vi "Pulse Parameters.vi"(0 "T1 Pulse Sequence":T19={"Preliminary Settings"={"Nº of Scans (ns)"=3, "Pulse Frequency"=10000000.0, "Nº of Vd"=3}, "Pulse Settings"={"Duration Signal P2"=20.0, "Power Level P2"=1023, "Phase P2"=90, "P2 Unit"=0, "Duration Signal P1"=20.0, "Power Level P1"=1023, "Phase P1"=90, "P1 Unit"=0}, "Acquisition Settings"={"Number Samples"=2000, "Time Between Points"=0.0, "Unit"=0}, "Delay Settings"={"Delay d1"=10.0, "Delay d2"=0.0, "d1 Unit"=0, "d2 Unit"=0, "Delay d30"=0.0, "d30 Unit"=0, "Vd Unit"=0, "Vd Values"="0"}} {"Delay Settings"."Vd Unit" items=["us", "ms"]; "Delay Settings"."d30 Unit" items=["us", "ms"]; "Delay Settings"."Delay d30" min=0.0 step=1.0; "Delay Settings"."d2 Unit" items=["us", "ms"]; "Delay Settings"."d1 Unit" items=["us", "ms"]; "Delay Settings"."Delay d2" min=0.0 step=1.0 format="%#_4g"; "Delay Settings"."Delay d1" min=0.0 step=1.0 format="%#_4g"; "Acquisition Settings"."Unit" items=["us", "ms"]; "Acquisition Settings"."Time Between Points" min=0.0 step=1.0; "Acquisition Settings"."Number Samples" step=1; "Pulse Settings"."P1 Unit" items=["us", "ms"]; "Pulse Settings"."Phase P1" max=270 step=90; "Pulse Settings"."Power Level P1" max=1023 step=1; "Pulse Settings"."Duration Signal P1" min=0.0 step=1.0 format="%#_4g"; "Pulse Settings"."P2 Unit" items=["us", "ms"]; "Pulse Settings"."Phase P2" max=270 step=90; "Pulse Settings"."Power Level P2" max=1023 step=1; "Pulse Settings"."Duration Signal P2" min=0.0 step=1.0 format="%#_4g"; "Preliminary Settings"."Nº of Vd" step=1; "Preliminary Settings"."Pulse Frequency" min=1.0 max=200000000.0 step=1000000.0 format="%^#_6e"; "Preliminary Settings"."Nº of Scans (ns)" step=1}, 1 "action":T20, 5 "90 Degree Pulse Sequence":T18={"Delay Settings"={"Delay d1"=10.0, "Delay d2"=0.0, "d1 Unit"=0, "d2 Unit"=0}, "Preliminary Settings"={"Nº of Scans (ns)"=3, "Pulse Frequency"=10000000.0}, "Pulse Settings"={"Duration Signal P1"=20.0, "Power Level"=1023, "Phase"=90, "P1 Units"=0}, "Acquisition Settings"={"Number Samples"=2000, "Time Between Points"=0.0, "Unit"=0}} {"Acquisition Settings"."Unit" items=["us", "ms"]; "Acquisition Settings"."Time Between Points" min=0.0 step=1.0; "Acquisition Settings"."Number Samples" step=1; "Pulse Settings"."P1 Units" items=["us", "ms"]; "Pulse Settings"."Phase" max=270 step=90; "Pulse Settings"."Power Level" max=1023 step=1; "Pulse Settings"."Duration Signal P1" min=0.0 step=1.0 format="%#_4g"; "Preliminary Settings"."Pulse Frequency" min=1.0 max=200000000.0 step=1000000.0 format="%^#_6e"; "Preliminary Settings"."Nº of Scans (ns)" step=1; "Delay Settings"."d2 Unit" items=["us", "ms"]; "Delay Settings"."d1 Unit" items=["us", "ms"]; "Delay Settings"."Delay d2" min=0.0 step=1.0 format="%#_4g"; "Delay Settings"."Delay d1" min=0.0 step=1.0 format="%#_4g"}, 7 "CPMG Pulse Sequence":T17={"Acquisition Settings"={"Number Samples"=2000, "Time Between Points"=0.0, "Unit"=0}, "Delay Settings"={"Delay d1"=10.0, "Delay d2"=0.0, "d1 Unit"=0, "d2 Unit"=0, "Delay d3"=0.0, "d3 Unit"=0, "Delay d4"=0.0, "d4 Unit"=0}, "Preliminary Settings"={"Nº of Scans (ns)"=3, "Pulse Frequency"=10000000.0, "Nº of Echoes (ne)"=3}, "Pulse Settings"={"Duration Signal P1"=20.0, "Power Level P1"=1023, "Phase P1"=90, "P1 Unit"=0, "Duration Signal P2"=20.0, "Power Level P2"=1023, "Phase P2"=90, "P2 Unit"=0}} {"Pulse Settings"."P2 Unit" items=["us", "ms"]; "Pulse Settings"."Phase P2" max=270 step=90; "Pulse Settings"."Power Level P2" max=1023 step=1; "Pulse Settings"."Duration Signal P2" min=0.0 step=1.0 format="%#_4g"; "Pulse Settings"."P1 Unit" items=["us", "ms"]; "Pulse Settings"."Phase P1" max=270 step=90; "Pulse Settings"."Power Level P1" max=1023 step=1; "Pulse Settings"."Duration Signal P1" min=0.0 step=1.0 format="%#_4g"; "Preliminary Settings"."Nº of Echoes (ne)" step=1; "Preliminary Settings"."Pulse Frequency" min=1.0 max=200000000.0 step=1000000.0 format="%^#_6e"; "Preliminary Settings"."Nº of Scans (ns)" step=1; "Delay Settings"."d4 Unit" items=["us", "ms"]; "Delay Settings"."Delay d4" min=0.0 step=1.0 format="%#_4g"; "Delay Settings"."d3 Unit" items=["us", "ms"]; "Delay Settings"."Delay d3" min=0.0 step=1.0 format="%#_4g"; "Delay Settings"."d2 Unit" items=["us", "ms"]; "Delay Settings"."d1 Unit" items=["us", "ms"]; "Delay Settings"."Delay d2" min=0.0 step=1.0 format="%#_4g"; "Delay Settings"."Delay d1" min=0.0 step=1.0 format="%#_4g"; "Acquisition Settings"."Unit" items=["us", "ms"]; "Acquisition Settings"."Time Between Points" min=0.0 step=1.0; "Acquisition Settings"."Number Samples" step=1}, 11 "error in":errorcluster) -> (4 "T1 Pulse settings Out":T9={"Preliminary Settings"={"Nº of Scans (ns)"=3, "Pulse Frequency"=10000000.0, "Nº of Vd"=3}, "Pulse Settings"={"Duration Signal P2"=20.0, "Power Level P2"=1023, "Phase P2"=90, "P2 Unit"=0, "Duration Signal P1"=20.0, "Power Level P1"=1023, "Phase P1"=90, "P1 Unit"=0}, "Acquisition Settings"={"Number Samples"=2000, "Time Between Points"=0.0, "Unit"=0}, "Delay Settings"={"Delay d1"=10.0, "Delay d2"=0.0, "d1 Unit"=0, "d2 Unit"=0, "Delay d30"=0.0, "d30 Unit"=0, "Vd Unit"=0, "Vd Values"="0"}} {"Delay Settings"."Vd Unit" items=["us", "ms"]; "Delay Settings"."d30 Unit" items=["us", "ms"]; "Delay Settings"."Delay d30" min=0.0 step=1.0; "Delay Settings"."d2 Unit" items=["us", "ms"]; "Delay Settings"."d1 Unit" items=["us", "ms"]; "Delay Settings"."Delay d2" min=0.0 step=1.0 format="%#_4g"; "Delay Settings"."Delay d1" min=0.0 step=1.0 format="%#_4g"; "Acquisition Settings"."Unit" items=["us", "ms"]; "Acquisition Settings"."Time Between Points" min=0.0 step=1.0; "Acquisition Settings"."Number Samples" step=1; "Pulse Settings"."P1 Unit" items=["us", "ms"]; "Pulse Settings"."Phase P1" max=270 step=90; "Pulse Settings"."Power Level P1" max=1023 step=1; "Pulse Settings"."Duration Signal P1" min=0.0 step=1.0 format="%#_4g"; "Pulse Settings"."P2 Unit" items=["us", "ms"]; "Pulse Settings"."Phase P2" max=270 step=90; "Pulse Settings"."Power Level P2" max=1023 step=1; "Pulse Settings"."Duration Signal P2" min=0.0 step=1.0 format="%#_4g"; "Preliminary Settings"."Nº of Vd" step=1; "Preliminary Settings"."Pulse Frequency" min=1.0 max=200000000.0 step=1000000.0 format="%^#_6e"; "Preliminary Settings"."Nº of Scans (ns)" step=1}, 6 "90 Degree Pulse settings out":T13={"Delay Settings"={"Delay d1"=10.0, "Delay d2"=0.0, "d1 Unit"=0, "d2 Unit"=0}, "Preliminary Settings"={"Nº of Scans (ns)"=3, "Pulse Frequency"=10000000.0}, "Pulse Settings"={"Duration Signal P1"=20.0, "Power Level"=1023, "Phase"=90, "P1 Units"=0}, "Acquisition Settings"={"Number Samples"=2000, "Time Between Points"=0.0, "Unit"=0}} {"Acquisition Settings"."Unit" items=["us", "ms"]; "Acquisition Settings"."Time Between Points" min=0.0 step=1.0; "Acquisition Settings"."Number Samples" step=1; "Pulse Settings"."P1 Units" items=["us", "ms"]; "Pulse Settings"."Phase" max=270 step=90; "Pulse Settings"."Power Level" max=1023 step=1; "Pulse Settings"."Duration Signal P1" min=0.0 step=1.0 format="%#_4g"; "Preliminary Settings"."Pulse Frequency" min=1.0 max=200000000.0 step=1000000.0 format="%^#_6e"; "Preliminary Settings"."Nº of Scans (ns)" step=1; "Delay Settings"."d2 Unit" items=["us", "ms"]; "Delay Settings"."d1 Unit" items=["us", "ms"]; "Delay Settings"."Delay d2" min=0.0 step=1.0 format="%#_4g"; "Delay Settings"."Delay d1" min=0.0 step=1.0 format="%#_4g"}, 8 "CPMG pulse settings Out":T5={"Acquisition Settings"={"Number Samples"=2000, "Time Between Points"=0.0, "Unit"=0}, "Delay Settings"={"Delay d1"=10.0, "Delay d2"=0.0, "d1 Unit"=0, "d2 Unit"=0, "Delay d3"=0.0, "d3 Unit"=0, "Delay d4"=0.0, "d4 Unit"=0}, "Preliminary Settings"={"Nº of Scans (ns)"=3, "Pulse Frequency"=10000000.0, "Nº of Echoes (ne)"=3}, "Pulse Settings"={"Duration Signal P1"=20.0, "Power Level P1"=1023, "Phase P1"=90, "P1 Unit"=0, "Duration Signal P2"=20.0, "Power Level P2"=1023, "Phase P2"=90, "P2 Unit"=0}} {"Pulse Settings"."P2 Unit" items=["us", "ms"]; "Pulse Settings"."Phase P2" max=270 step=90; "Pulse Settings"."Power Level P2" max=1023 step=1; "Pulse Settings"."Duration Signal P2" min=0.0 step=1.0 format="%#_4g"; "Pulse Settings"."P1 Unit" items=["us", "ms"]; "Pulse Settings"."Phase P1" max=270 step=90; "Pulse Settings"."Power Level P1" max=1023 step=1; "Pulse Settings"."Duration Signal P1" min=0.0 step=1.0 format="%#_4g"; "Preliminary Settings"."Nº of Echoes (ne)" step=1; "Preliminary Settings"."Pulse Frequency" min=1.0 max=200000000.0 step=1000000.0 format="%^#_6e"; "Preliminary Settings"."Nº of Scans (ns)" step=1; "Delay Settings"."d4 Unit" items=["us", "ms"]; "Delay Settings"."Delay d4" min=0.0 step=1.0 format="%#_4g"; "Delay Settings"."d3 Unit" items=["us", "ms"]; "Delay Settings"."Delay d3" min=0.0 step=1.0 format="%#_4g"; "Delay Settings"."d2 Unit" items=["us", "ms"]; "Delay Settings"."d1 Unit" items=["us", "ms"]; "Delay Settings"."Delay d2" min=0.0 step=1.0 format="%#_4g"; "Delay Settings"."Delay d1" min=0.0 step=1.0 format="%#_4g"; "Acquisition Settings"."Unit" items=["us", "ms"]; "Acquisition Settings"."Time Between Points" min=0.0 step=1.0; "Acquisition Settings"."Number Samples" step=1}, 10 "CMD STR Array":string[](array[string]), 12 "T1 set times":T15={"Real Time P1"=20.011287076734621636, "Real Time P2"=20.011287076734621636, "Real Time d1"=10.036661125207804438, "Real Time d2"=1.462, "Real Time d30"=1.462, "Real Time AQS"=0.73746299999999999998}, 13 "CPMG Set Times":T14={"Real Time d4"=69.971913553241751126, "Real Time d3"=50.022661650188109273, "Real Time P2"=39.96053897978825603, "Real Time d2"=29.985913028261440076, "Real Time P1"=20.011287076734621636, "Real Time d1"=10.036661125207804438, "Real Time AQS"=0.73746299999999999998}, 14 "Set Time 90 Degree Pulse":T16, 15 "error out":errorcluster)   [LabVIEW 2011]
uses:
  Pulse Parameters.ctl
  Controls/Full_T1 Degree Pulse Settings.ctl
  Controls/T1_Preliminary Settings.ctl
  Controls/T1_Pulse Settings.ctl
  Controls/Acquisition Settings.ctl
  Controls/T1_Delay Settings.ctl
  Controls/Full_90 Degree Pulse Settings.ctl
  Controls/90D_Delay Settings.ctl
  Controls/90D_Preliminary Settings.ctl
  Controls/90D_Pulse Settings.ctl
  Controls/Full_CPMG Degree Pulse Settings.ctl
  Controls/CPMG_Delay Settings.ctl
  Controls/CPMG_Preliminary Settings.ctl
  Controls/CPMG_Pulse Settings.ctl
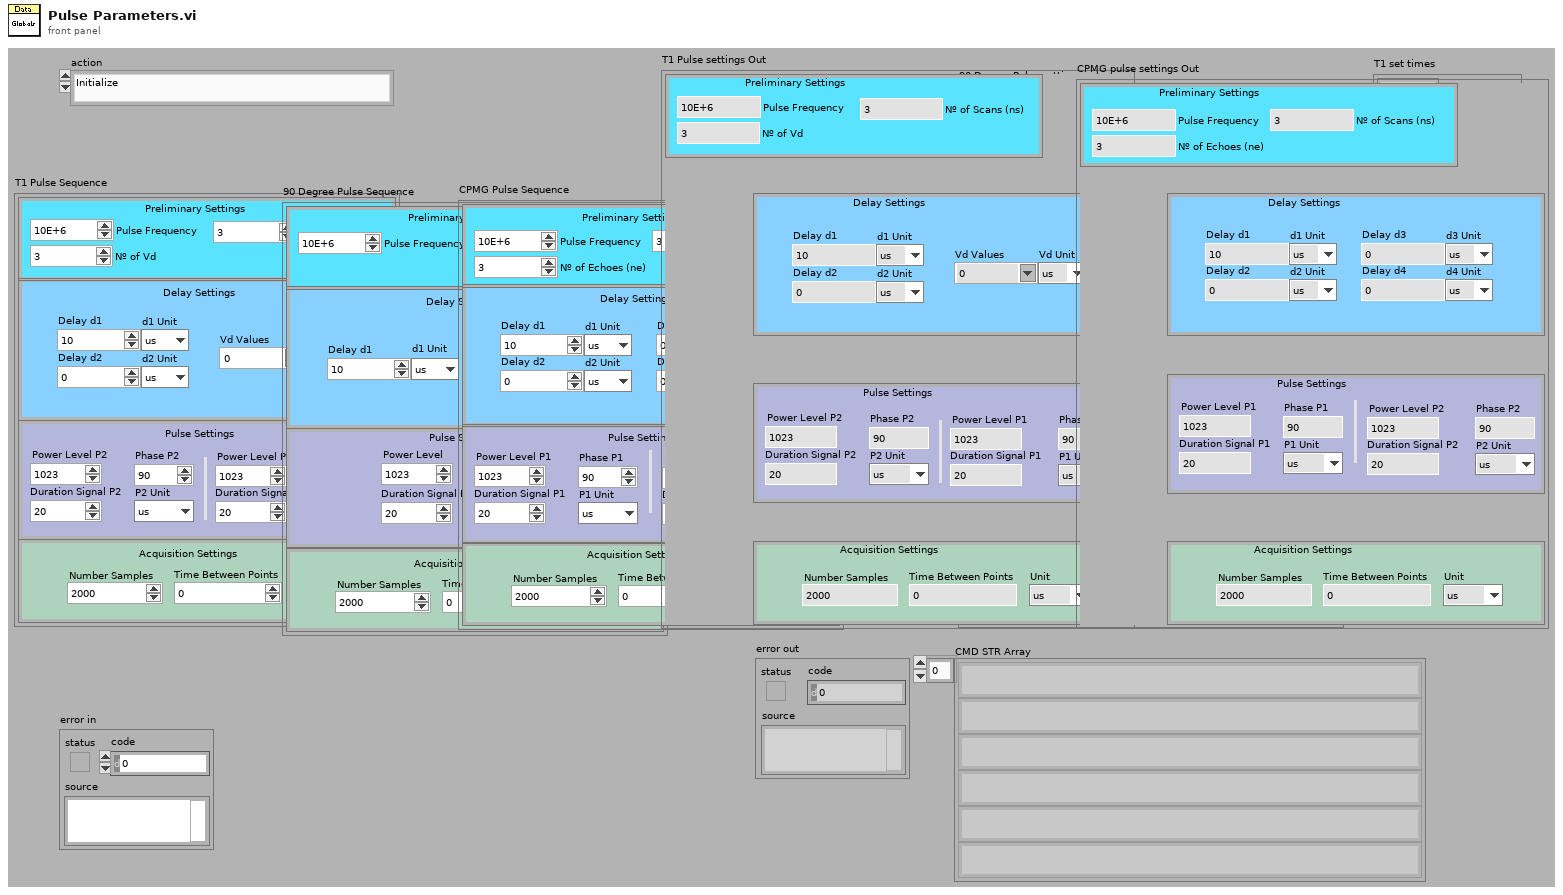
[diagram p1: front panel]
types:
  T1 = typedef "Acquisition Settings.ctl" = cluster{"Number Samples":u16, "Time Between Points":dbl, "Unit":u8}
  T2 = typedef "CPMG_Delay Settings.ctl" = cluster{"Delay d1":dbl, "Delay d2":dbl, "d1 Unit":u8, "d2 Unit":u8, "Delay d3":dbl, "d3 Unit":u8, "Delay d4":dbl, "d4 Unit":u8}
  T3 = typedef "CPMG_Preliminary Settings.ctl" = cluster{"Nº of Scans (ns)":u16, "Pulse Frequency":dbl, "Nº of Echoes (ne)":u16}
  T4 = typedef "CPMG_Pulse Settings.ctl" = cluster{"Duration Signal P1":dbl, "Power Level P1":u16, "Phase P1":u16, "P1 Unit":u8, "Duration Signal P2":dbl, "Power Level P2":u16, "Phase P2":u16, "P2 Unit":u8}
  T5 = cluster{"Acquisition Settings":T1, "Delay Settings":T2, "Preliminary Settings":T3, "Pulse Settings":T4}
  T6 = typedef "T1_Preliminary Settings.ctl" = cluster{"Nº of Scans (ns)":u16, "Pulse Frequency":dbl, "Nº of Vd":u16}
  T7 = typedef "T1_Pulse Settings.ctl" = cluster{"Duration Signal P2":dbl, "Power Level P2":u16, "Phase P2":u16, "P2 Unit":u8, "Duration Signal P1":dbl, "Power Level P1":u16, "Phase P1":u16, "P1 Unit":u8}
  T8 = typedef "T1_Delay Settings.ctl" = cluster{"Delay d1":dbl, "Delay d2":dbl, "d1 Unit":u8, "d2 Unit":u8, "Delay d30":dbl, "d30 Unit":u8, "Vd Unit":u8, "Vd Values":string}
  T9 = cluster{"Preliminary Settings":T6, "Pulse Settings":T7, "Acquisition Settings":T1, "Delay Settings":T8}
  T10 = typedef "90D_Delay Settings.ctl" = cluster{"Delay d1":dbl, "Delay d2":dbl, "d1 Unit":u8, "d2 Unit":u8}
  T11 = typedef "90D_Preliminary Settings.ctl" = cluster{"Nº of Scans (ns)":u16, "Pulse Frequency":dbl}
  T12 = typedef "90D_Pulse Settings.ctl" = cluster{"Duration Signal P1":dbl, "Power Level":u16, "Phase":u16, "P1 Units":u8}
  T13 = cluster{"Delay Settings":T10, "Preliminary Settings":T11, "Pulse Settings":T12, "Acquisition Settings":T1}
  T14 = cluster{"Real Time d4":ext, "Real Time d3":ext, "Real Time P2":ext, "Real Time d2":ext, "Real Time P1":ext, "Real Time d1":ext, "Real Time AQS":ext}
  T15 = cluster{"Real Time P1":ext, "Real Time P2":ext, "Real Time d1":ext, "Real Time d2":ext, "Real Time d30":ext, "Real Time AQS":ext}
  T16 = cluster{"D1 Real Time":ext, "D2 Real Time":ext, "P1 Real Time":ext, "AQS Real Time":ext}
  T17 = typedef "Full_CPMG Degree Pulse Settings.ctl" = cluster{"Acquisition Settings":T1, "Delay Settings":T2, "Preliminary Settings":T3, "Pulse Settings":T4}
  T18 = typedef "Full_90 Degree Pulse Settings.ctl" = cluster{"Delay Settings":T10, "Preliminary Settings":T11, "Pulse Settings":T12, "Acquisition Settings":T1}
  T19 = typedef "Full_T1 Degree Pulse Settings.ctl" = cluster{"Preliminary Settings":T6, "Pulse Settings":T7, "Acquisition Settings":T1, "Delay Settings":T8}
  T20 = typedef "Pulse Parameters.ctl" = enum16{"Initialize", "Set T1 Pulse Settings", "Set 90 Degree Pulse Settings", "Set CPMG Pulse Settings", "Get T1 Settings", "Get CPMG Settings", "Get 90 Degree Settings"}
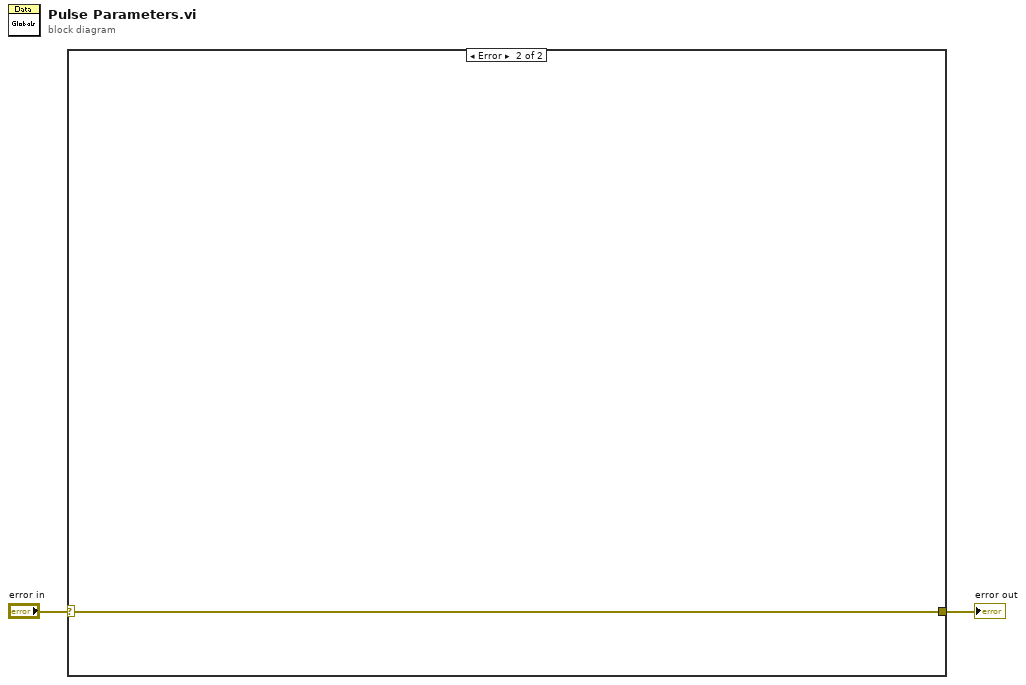
[diagram p0: block diagram]
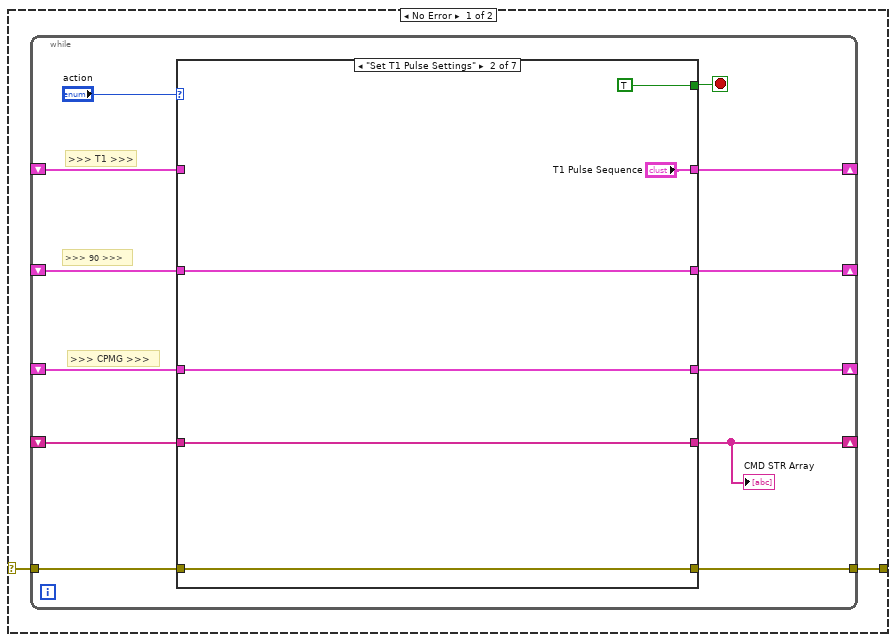
[diagram p2: hidden frame]
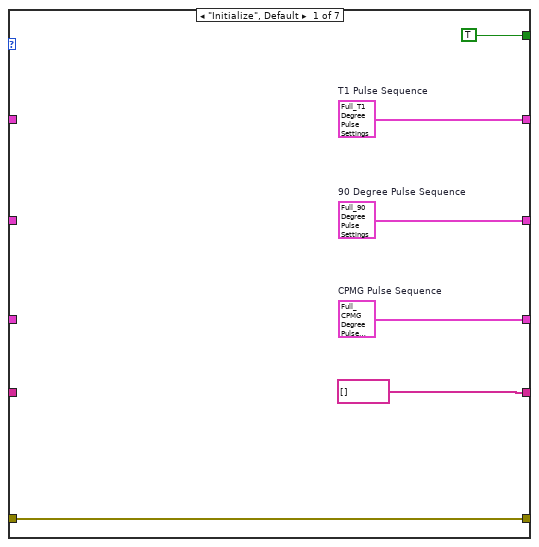
[diagram p3: hidden frame]
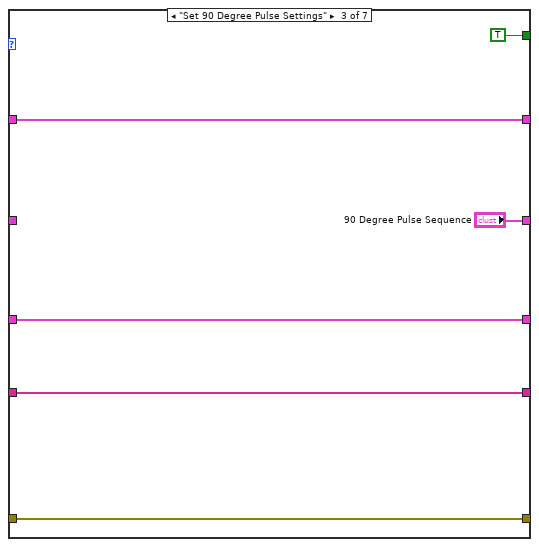
[diagram p4: hidden frame]
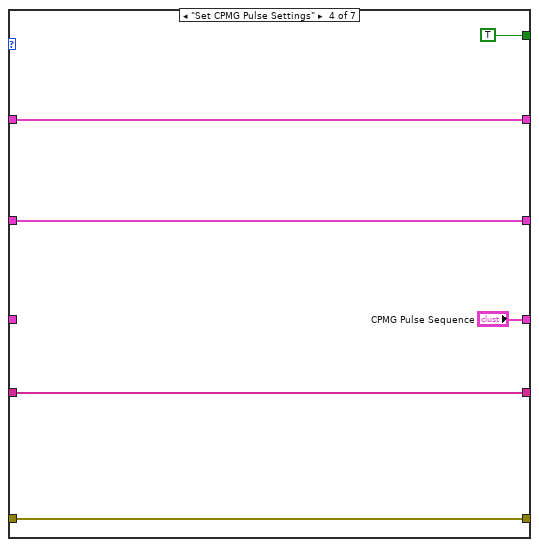
[diagram p5: hidden frame]
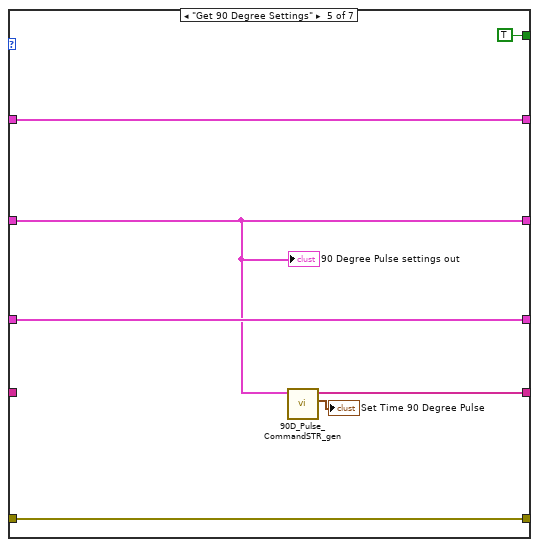
[diagram p6: hidden frame]
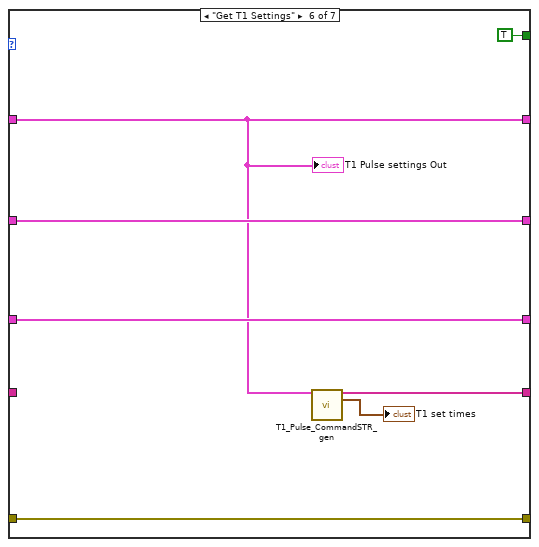
[diagram p7: hidden frame]
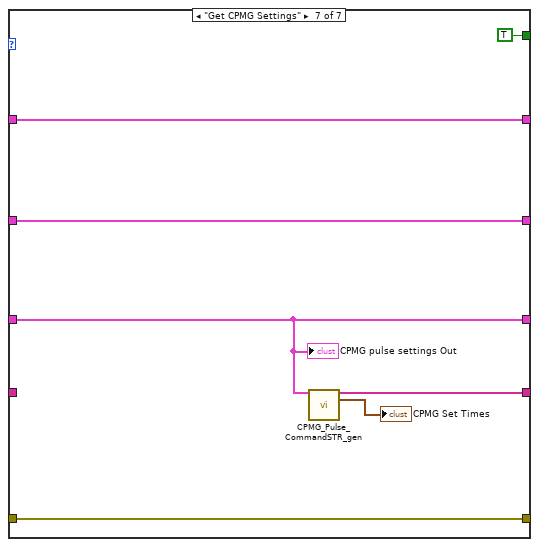
[diagram p8: hidden frame]
diagram:
  n1 = case shown="Error" "error in" {
    selector: "error in" -> [w4 w62]
    tunnel: [w3 w62] -> w1
    frame No Error {
      n2 = while {
        tunnel: w4 -> [w15]
        tunnel: [w14] -> w3
        shift-right: [w12] -> _
        shift-left: _ -> [w11]
        shift-right: [w10] -> _
        shift-left: _ -> [w9]
        shift-right: [w8] -> _
        shift-left: _ -> [w7]
        shift-right: [w6] -> _
        shift-left: _ -> [w5]
        stop <- w13 stop-if-true
        # ">>> CPMG >>>"
        # ">>> 90 >>>"
        # ">>> T1 >>>"
        n3 = case shown="\"Set T1 Pulse Settings\"" "action" {
          tunnel: w15 -> [w21 w28 w31 w37 w41 w49 w55]
          tunnel: [w21 w28 w31 w37 w41 w49 w55] -> w14
          tunnel: [TRUE TRUE TRUE TRUE TRUE TRUE TRUE] -> w13
          tunnel: [w20 "T1 Pulse Sequence" w34 w40 w47 w48 w61] -> w12
          tunnel: w11 -> [_ _ w34 w40 w47 w48 w61]
          tunnel: [w19 w25 "90 Degree Pulse Sequence" w39 w42 w54 w60] -> w10
          tunnel: w9 -> [_ w25 _ w39 w42 w54 w60]
          tunnel: [w18 w24 w32 "CPMG Pulse Sequence" w46 w53 w56] -> w8
          tunnel: w7 -> [_ w24 w32 _ w46 w53 w56]
          tunnel: [string[] [] w23 w29 w35 w44 w52 w59] -> w6
          tunnel: w5 -> [_ w23 w29 w35 _ _ _]
          frame "Initialize", Default {
            w18 = T17 {"Acquisition Settings"={"Number Samples"=0, "Time Between Points"=0.0, "Unit"=0}, "Delay Settings"={"Delay d1"=0.0, "Delay d2"=0.0, "d1 Unit"=0, "d2 Unit"=0, "Delay d3"=0.0, "d3 Unit"=0, "Delay d4"=0.0, "d4 Unit"=0}, "Preliminary Settings"={"Nº of Scans (ns)"=3, "Pulse Frequency"=10000000.0, "Nº of Echoes (ne)"=3}, "Pulse Settings"={"Duration Signal P1"=0.0, "Power Level P1"=0, "Phase P1"=0, "P1 Unit"=0, "Duration Signal P2"=0.0, "Power Level P2"=0, "Phase P2"=0, "P2 Unit"=0}}  # CPMG Pulse Sequence
            w19 = T18 {"Delay Settings"={"Delay d1"=0.0, "Delay d2"=0.0, "d1 Unit"=0, "d2 Unit"=0}, "Preliminary Settings"={"Nº of Scans (ns)"=3, "Pulse Frequency"=10000000.0}, "Pulse Settings"={"Duration Signal P1"=0.0, "Power Level"=0, "Phase"=0, "P1 Units"=0}, "Acquisition Settings"={"Number Samples"=0, "Time Between Points"=0.0, "Unit"=0}}  # 90 Degree Pulse Sequence
            w20 = T19 {"Preliminary Settings"={"Nº of Scans (ns)"=3, "Pulse Frequency"=10000000.0, "Nº of Vd"=3}, "Pulse Settings"={"Duration Signal P2"=0.0, "Power Level P2"=0, "Phase P2"=0, "P2 Unit"=0, "Duration Signal P1"=0.0, "Power Level P1"=0, "Phase P1"=0, "P1 Unit"=0}, "Acquisition Settings"={"Number Samples"=0, "Time Between Points"=0.0, "Unit"=0}, "Delay Settings"={"Delay d1"=0.0, "Delay d2"=0.0, "d1 Unit"=0, "d2 Unit"=0, "Delay d30"=0.0, "d30 Unit"=0, "Vd Unit"=0, "Vd Values"=""}}  # T1 Pulse Sequence
          }
          frame "Set T1 Pulse Settings" {
          }
          frame "Set 90 Degree Pulse Settings" {
          }
          frame "Set CPMG Pulse Settings" {
          }
          frame "Get 90 Degree Settings" {
            n4 = call "90D_Pulse_CommandSTR_gen.vi"("90 Degree Pulse Sequence"=w42) -> ("90 Set Times"=→"Set Time 90 Degree Pulse":T16, "CMD STR Array"=w44:string[])  [unwired: 9 in]
            "90 Degree Pulse settings out" <- w42
          }
          frame "Get T1 Settings" {
            n5 = call "T1_Pulse_CommandSTR_gen.vi"("T1 Pulse Sequence"=w48) -> ("Array"=w52:string[], "T1 set times"=→"T1 set times":T15)  [unwired: 12 in, 1 out]
            "T1 Pulse settings Out" <- w48
          }
          frame "Get CPMG Settings" {
            n6 = call "CPMG_Pulse_CommandSTR_gen.vi"("CPMG Pulse Sequence"=w56) -> ("CMD STR Array"=w59:string[], "CPMG Set Times"=→"CPMG Set Times":T14)  [unwired: 13 in]
            "CPMG pulse settings Out" <- w56
          }
        }
        "CMD STR Array" <- w6
      }
    }
    frame Error {
    }
  }
  "error out" <- w1
